vi "New_Magazine_Set.vi"() -> ()   [LabVIEW 2019]
uses:
  New_Magazine_Globals.vi
  New_Magazine_Cluster.ctl
  New_Magazine_Control_States.ctl
panel:
  in  "Flywheel Spun-up":dbl
  in  "Spindexer Spun-up":dbl
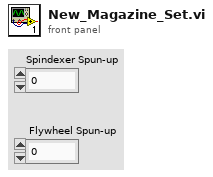
[diagram p1: front panel]
types:
  T1 = typedef "New_Magazine_Cluster.ctl" = cluster{"Control_States":T2, "Firing":bool, "Throttle":dbl, "Spinning Up":bool, "Off":bool}
  T2 = typedef "New_Magazine_Control_States.ctl" = enum16{"Up", "Down", "Manual", "Fire", "Spinning Up"}
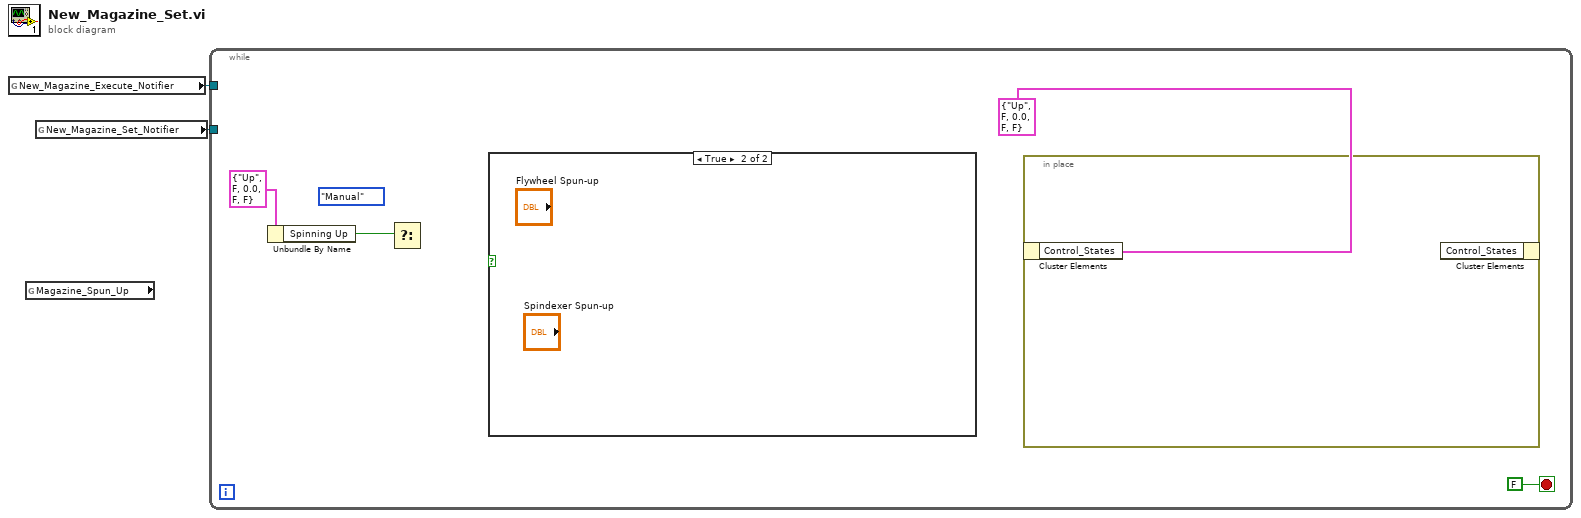
[diagram p0: block diagram]
diagram:
  n1 = global read "New_Magazine_Globals.vi" "New_Magazine_Execute_Notifier"() -> (w2:refnum<notifier>)
  n2 = global read "New_Magazine_Globals.vi" "Magazine_Spun_Up"() -> ()  [unwired: 1 out]
  n3 = global read "New_Magazine_Globals.vi" "New_Magazine_Set_Notifier"() -> (w1:refnum<notifier>)
  n4 = while {
    tunnel: w2 -> [_]
    tunnel: w1 -> [_]
    stop <- FALSE stop-if-true
    (unwired) enum16{"Up", "Down", "Manual", "Fire"}."Manual" ("Control_States")
    n5 = Unbundle By Name(T1 {"Control_States"=enum."Up", "Firing"=FALSE, "Throttle"=0.0, "Spinning Up"=FALSE, "Off"=FALSE} ("New_Magazine")) -> ("Spinning Up"=w3:bool)
    n6 = Select(s=w3) -> ()  [unwired: 2 in, 1 out]
    n7 = case shown="True" {
      selector: _ -> [_ _]
      frame False {
      }
      frame True {
      }
    }
    n8 = in-place {
      n9 = in-place-cluster #1(T1 {"Control_States"=enum."Up", "Firing"=FALSE, "Throttle"=0.0, "Spinning Up"=FALSE, "Off"=FALSE} ("New_Magazine")) -> ()  [unwired: 1 out]
      n10 = in-place-cluster #1() -> ()  [unwired: 1 in, 1 out]
    }
  }
